vi "Digitizer Aperture.vi"(0 "VISA resource name":refnum<visa-resource-name>="USB0::0x05E6::0x2461::04090176::INSTR", 5 "Digitize Function (Voltage)":u16(ring) items=["Voltage", "Current"], 7 "Aperture (.000001)":dbl=1e-05 format="%#_6f", 9 "Auto Aperture":bool=TRUE, 11 "error in (no error)":errorcluster) -> (4 "VISA resource name out":refnum<visa-resource-name>="USB0::0x05E6::0x2461::04090176::INSTR", 15 "error out":errorcluster)   [LabVIEW 2018, in "Keithley 2450.lvlib"]
doc: "This command determines the aperture setting for the selected function.\n\n<B>The Digitizer Voltage and Digitizer Current functions are only compatible with the 2461.</B>"
uses:
  <instrlib>/Keithley 2450/Keithley 2450.lvlib
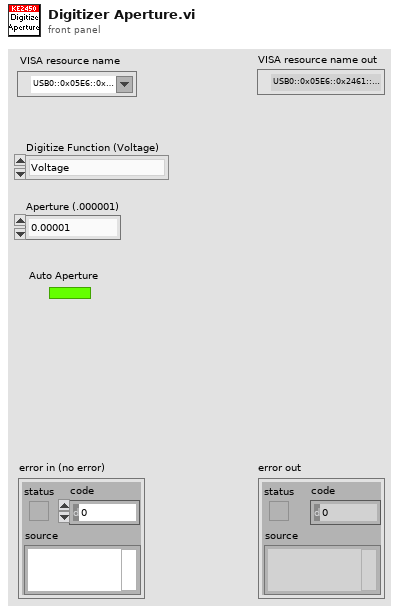
[diagram p1: front panel]
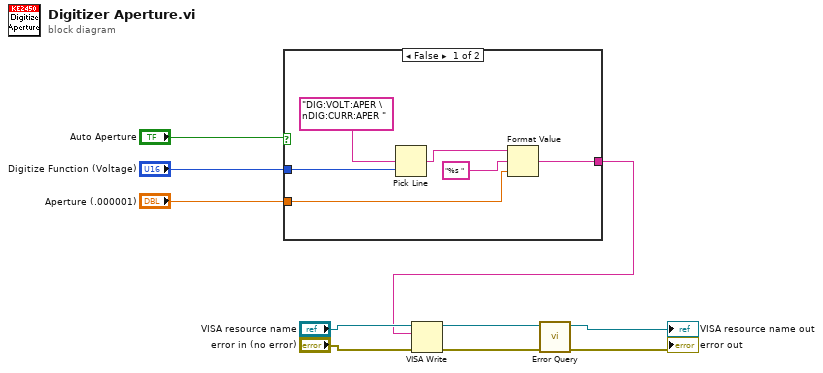
[diagram p0: block diagram]
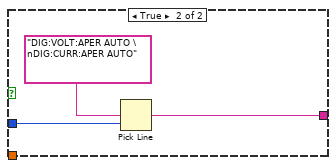
[diagram p2: hidden frame]
diagram:
  n1 = case shown="False" "Auto Aperture" {
    tunnel: "Digitize Function (Voltage)" -> [w16 w19]
    tunnel: "Aperture (.000001)" -> [w14 _]
    tunnel: [w11 w17] -> w1
    frame False {
      n2 = Pick Line(multi-line string="DIG:VOLT:APER \nDIG:CURR:APER ", line index=w16) -> (output string=w13:string)  [unwired: 1 in]
      n3 = Format Value(string ("")=w13, format string="%s ", value (0)=w14) -> (output string=w11:string)
    }
    frame True {
      n4 = Pick Line(multi-line string="DIG:VOLT:APER AUTO \nDIG:CURR:APER AUTO", line index=w19) -> (output string=w17:string)  [unwired: 1 in]
    }
  }
  n5 = VISA Write(VISA resource name="VISA resource name", write buffer=w1, error in (no error)="error in (no error)") -> (VISA resource name out=w6:refnum<visa-resource-name>, error out=w5:errorcluster)  [unwired: 1 out]
  n6 = call <instrlib>:"Error Query.vi"("error in (no error)"=w5, "VISA resource name"=w6) -> ("error out"=→"error out":errorcluster, "VISA resource name out"=→"VISA resource name out":refnum<visa-resource-name>)  [unwired: 8 out]
